vi "Stop Core.vi"(10 "final error code":i32, 11 "ViewableActor in":refnum<class "ViewableActor.lvclass">) -> (3 "ViewableActor out":refnum<class "ViewableActor.lvclass">)   [LabVIEW 2020, in "ViewableActor.lvlib" / "ViewableActor.lvclass"]
doc: "(<B>Filename</B>: Actor Framework.lvlib:Actor.lvclass:Stop Core.vi)\n\nDefines what the actor does before it stops. Use the <B>final error code</B> input to determine whether the actor shut down in response to an error.\n\nBy default, this method does nothing. A descendant class may override it to define behavior, such as shutting down any processes the actor initiated in its override of the Actor Core method."
uses:
  ViewableActor.lvclass
  ViewableActor.lvclass/ViewableActor.ctl
  Read Actor Name.vi
  Read UI VI Ref.vi
  Read SubPanel Ref.vi
  Read Stop Event.vi
  <vilib>/Utility/config.llb/Write Key (I32).vi
  <vilib>/ActorFramework/Actor/Actor.lvclass
  <vilib>/Utility/config.llb/NI_LVConfig.lvlib
  ViewableActor.lvlib
  C:/Program Files (x86)/National Instruments/LabVIEW 2020/vi.lib/ActorFramework/Actor/Actor.lvclass
  C:/Users/AlexK/work/LabVIEW Programme/POLARIS Active Stretcher_LV2020/Submodules/Viewable Actor/ViewableActor/ViewableActor.lvclass
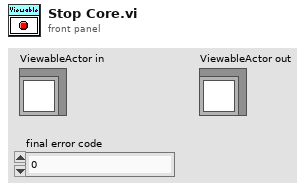
[diagram p1: front panel]
types:
  T1 = typedef "LVRectTypeDef.ctl" = cluster{"Left":i16, "Top":i16, "Right":i16, "Bottom":i16}
  T2 = typedef "NI_LVConfig.lvlib/Config Data RefNum.ctl" = refnum<k1>
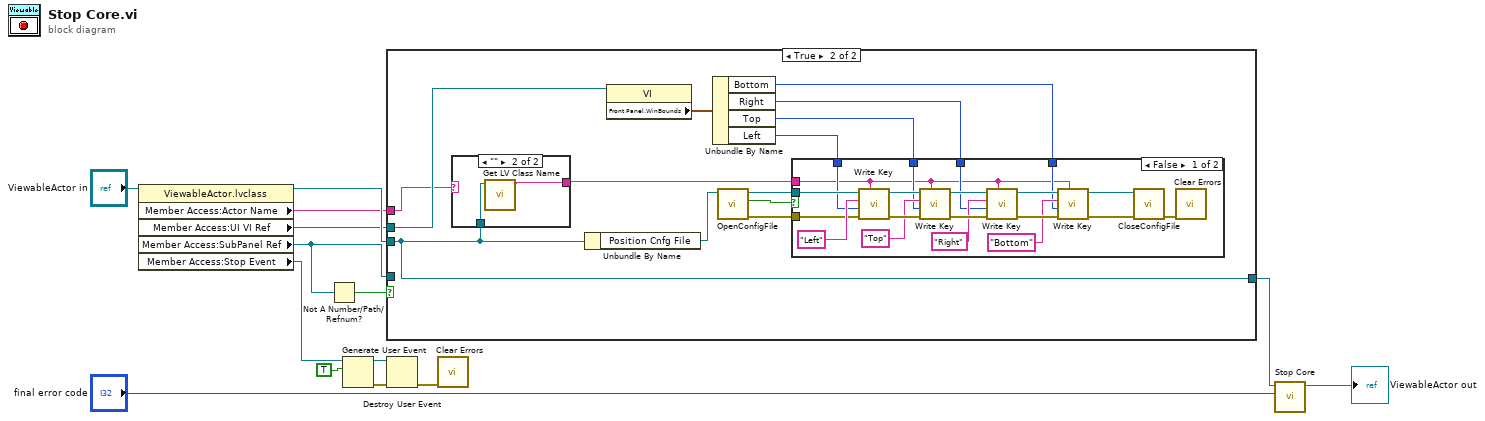
[diagram p0: block diagram]
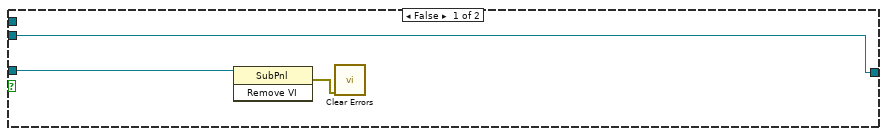
[diagram p2: hidden frame]
diagram:
  n1 = property class="ViewableActor.lvclass"(reference="ViewableActor in") -> (reference out=w4:refnum<class "ViewableActor.lvclass">, "Member Access:Actor Name"=w1:string, "Member Access:UI VI Ref"=w2:refnum<vi>, "Member Access:SubPanel Ref"=w8:refnum<vi>, "Member Access:Stop Event"=w3:refnum<user-event>)  [unwired: 1 in, 1 out]
  n2 = Not A Number/Path/Refnum?(number/path/refnum=w8) -> (NaN/Path/Refnum?=w9:bool)
  n3 = Generate User Event(user event=w3, event data cluster=TRUE ("event data")) -> (user event out=w11:refnum<user-event>, error out=w10:errorcluster)  [unwired: 2 in]
  n4 = case shown="True" w9 {
    tunnel: w8 -> [w17 _]
    tunnel: w2 -> [_ w30]
    tunnel: [w15 w20] -> w5
    tunnel: w4 -> [w15 w20]
    tunnel: w1 -> [_ w21]
    frame False {
      n5 = invoke class="SubPnl" method="Remove VI"(reference=w17) -> (error out=w16:errorcluster)  [unwired: 2 in, 2 out]
      n6 = call <vilib>:"Clear Errors.vi"("error in (no error)"=w16) -> ()  [unwired: 5 in, 2 out]
    }
    frame True {
      n7 = case shown="\"\"" w21 {
        selector: w21 -> [w51 _]
        tunnel: w20 -> [_ w53]
        tunnel: [w51 w52] -> w19
        frame Default {
        }
        frame "" {
          n8 = call <vilib>:"Get LV Class Name.vi"("object"=w53) -> ("class name"=w52:string)  [unwired: 9 in, 1 out]
        }
      }
      n9 = Unbundle By Name(w20) -> ("Position Cnfg File"=w27:path)
      n10 = property class="VI"(reference=w30) -> ("Front Panel.WinBounds"=w26:T1)  [unwired: 1 in, 2 out]
      n11 = Unbundle By Name(w26) -> ("Bottom"=w25:i16, "Right"=w24:i16, "Top"=w23:i16, "Left"=w22:i16)
      n12 = call "OpenConfigFile.vi"("configuration file path"=w27) -> ("error out"=w29:errorcluster, "timeout"=w18:bool, "refnum"=w28:T2)  [unwired: 8 in]
      n13 = case shown="False" w18 {
        tunnel: w29 -> [w40 _]
        tunnel: w28 -> [w39 _]
        tunnel: w25 -> [w35 _]
        tunnel: w24 -> [w34 _]
        tunnel: w23 -> [w33 _]
        tunnel: w22 -> [w32 _]
        tunnel: w19 -> [w31 _]
        frame False {
          n14 = call-poly <vilib>:"Write Key.vi"("section"=w31, "error in (no error)"=w40, "value"=w32, "key"="Left", "refnum"=w39) -> ("error out"=w42:errorcluster, "refnum out"=w41:T2)  [unwired: 4 in, 1 out]
          n15 = call-poly <vilib>:"Write Key.vi"("section"=w31, "error in (no error)"=w42, "value"=w33, "key"="Top", "refnum"=w41) -> ("error out"=w44:errorcluster, "refnum out"=w43:T2)  [unwired: 4 in, 1 out]
          n16 = call-poly <vilib>:"Write Key.vi"("section"=w31, "error in (no error)"=w44, "value"=w34, "key"="Right", "refnum"=w43) -> ("error out"=w46:errorcluster, "refnum out"=w45:T2)  [unwired: 4 in, 1 out]
          n17 = call-poly <vilib>:"Write Key.vi"("section"=w31, "error in (no error)"=w46, "value"=w35, "key"="Bottom", "refnum"=w45) -> ("error out"=w48:errorcluster, "refnum out"=w47:T2)  [unwired: 4 in, 1 out]
          n18 = call "CloseConfigFile.vi"("error in (no error)"=w48, "refnum"=w47) -> ("error out"=w50:errorcluster)  [unwired: 8 in, 1 out]
          n19 = call <vilib>:"Clear Errors.vi"("error in (no error)"=w50) -> ()  [unwired: 5 in, 2 out]
        }
        frame True {
        }
      }
    }
  }
  n20 = Destroy User Event(user event=w11, error in=w10) -> (error out=w7:errorcluster)
  n21 = call <vilib>:"Clear Errors.vi"("error in (no error)"=w7) -> ()  [unwired: 5 in, 2 out]
  n22 = call-parent "Stop Core.vi"("final error code"="final error code", "Actor in"=w5) -> ("Actor out"=→"ViewableActor out":refnum<class "ViewableActor.lvclass">)  [unwired: 9 in]
